vi "launcher.vi"() -> ()   [LabVIEW 2019]
uses:
  UI Actor/UI Actor.lvclass
  C:/Program Files (x86)/National Instruments/LabVIEW 2019/vi.lib/ActorFramework/Actor/Actor.lvclass
  UI Actor/UI Actor.lvclass/UI Actor.ctl
  UI Actor/Write Coins.vi
  UI Actor/Write Productos.vi
  <vilib>/ActorFramework/Actor/Actor.lvclass
panel:
  in  "Productos":enum16{"Coca", "Nestle"}(ring)
  in  "Coins":enum16{"MXN", "USD", ""}(ring)
  in  "error in (no error)":errorcluster
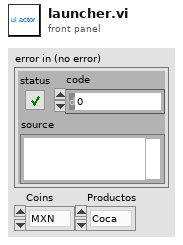
[diagram p1: front panel]
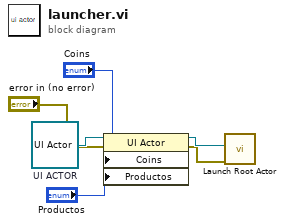
[diagram p0: block diagram]
diagram:
  w6 = refnum<class "UI Actor.lvclass"> refnum  # UI ACTOR
  n1 = property class="UI Actor"(reference=w6, error in="error in (no error)", "Coins"="Coins", "Productos"="Productos") -> (reference out=w5:refnum<class "UI Actor.lvclass">, error out=w3:errorcluster)
  n2 = call <vilib>:"Launch Root Actor.vi"("error in (no error)"=w3, "Actor"=w5) -> ()  [unwired: 8 in, 2 out]
